vi "Active.vi"(7 "FGV_mods":T1=enum."get", 8 "Error In":errorcluster, 11 "value":bool) -> (0 "Error Out":errorcluster, 3 "active":bool)   [LabVIEW 2016]
uses:
  Tools/variable_acess_mods.ctl
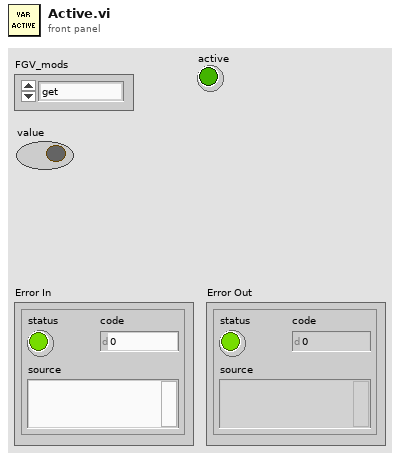
[diagram p1: front panel]
types:
  T1 = typedef "variable_acess_mods.ctl" = enum16{"init", "set", "get"}
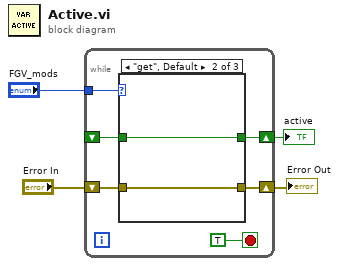
[diagram p0: block diagram]
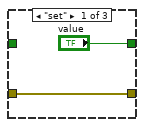
[diagram p2: hidden frame]
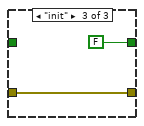
[diagram p3: hidden frame]
diagram:
  n1 = while {
    tunnel: "FGV_mods" -> [w9]
    shift-right: [w8] -> w1
    shift-left: _ -> [w7]
    shift-right: [w5] -> w2
    shift-left: "Error In" -> [w6]
    stop <- TRUE stop-if-true
    n2 = case shown="\"get\", Default" w9 {
      tunnel: ["value" w14 FALSE] -> w8
      tunnel: w7 -> [_ w14 _]
      tunnel: w6 -> [w12 w13 w15]
      tunnel: [w12 w13 w15] -> w5
      frame "set" {
      }
      frame "get", Default {
      }
      frame "init" {
      }
    }
  }
  "Error Out" <- w2
  "active" <- w1
